vi "Move Motors Y.vi"() -> ()   [LabVIEW 2014]
panel:
  in  "Current Motor Position past home (um)":string
  out "Motor XY After Moving":string
  in  "Camera Resolution X":i64
  in  "pix/micron":dbl
  in  "XY Mouse Position":string
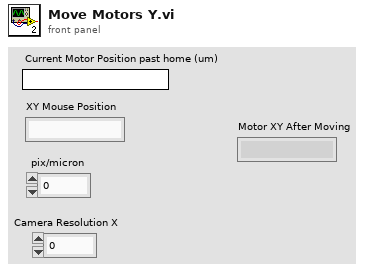
[diagram p1: front panel]
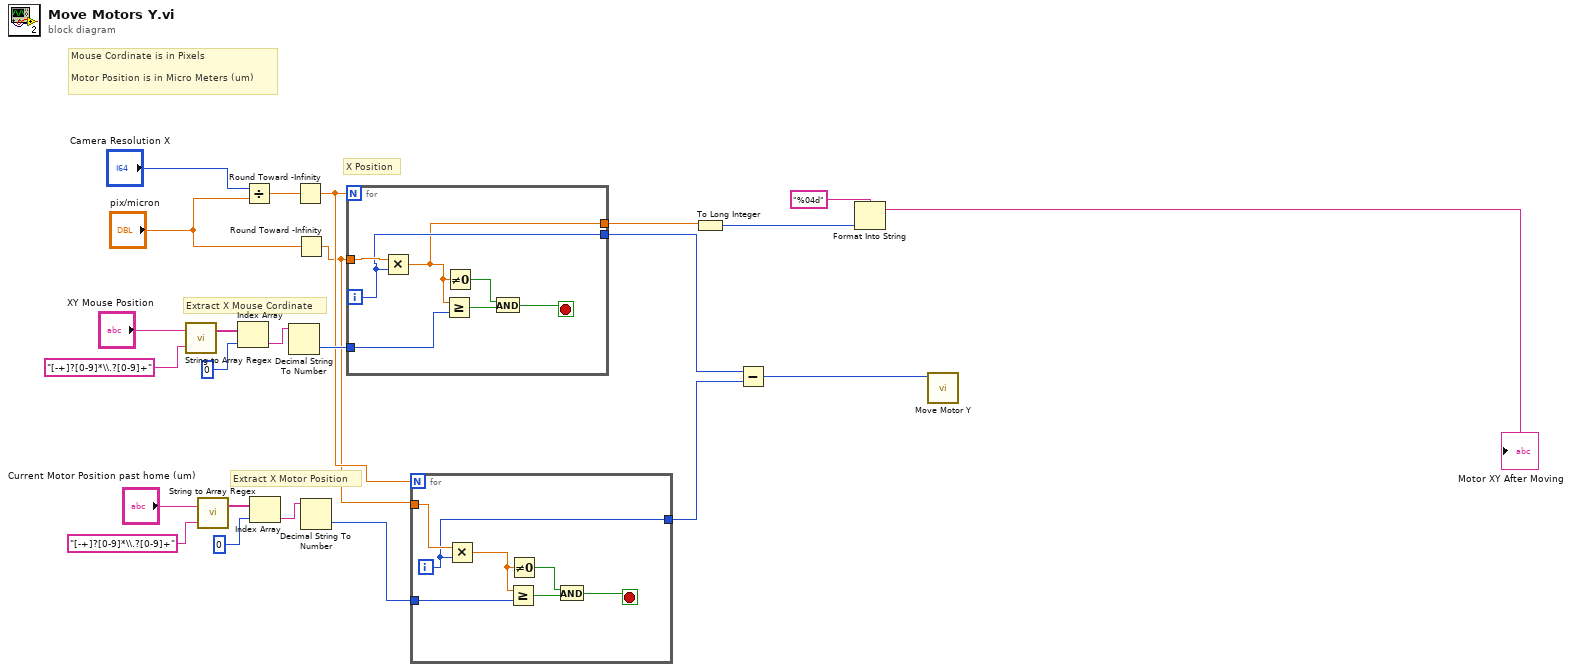
[diagram p0: block diagram]
diagram:
  # "Extract X Motor Position"
  # "Mouse Cordinate is in Pixels\n\nMotor Position is in Micro Meters (um)"
  # "Extract X Mouse Cordinate"
  # "X Position"
  n1 = call "String to Array Regex.vi"("Regex"="[-+]?[0-9]*\\.?[0-9]+", "Message"="XY Mouse Position") -> ("String to Array"=w20:string[])  [unwired: 1 in]
  n2 = call "String to Array Regex.vi"("Regex"="[-+]?[0-9]*\\.?[0-9]+", "Message"="Current Motor Position past home (um)") -> ("String to Array"=w13:string[])  [unwired: 1 in]
  n3 = Index Array(array=w20, index=0) -> (element=w17:string)
  n4 = Divide(x="Camera Resolution X", y="pix/micron") -> (x/y=w23:dbl)
  n5 = Index Array(array=w13, index=0) -> (element=w11:string)
  n6 = Decimal String To Number(string=w17) -> (number=w18:i32)  [unwired: 2 in, 1 out]
  n7 = Round Toward -Infinity(1:w23) -> (0:w8:dbl)
  n8 = Round Toward -Infinity(1:"pix/micron") -> (0:w7:dbl)
  n9 = Decimal String To Number(string=w11) -> (number=w5:i32)  [unwired: 2 in, 1 out]
  n10 = for {
    N: w8 -> [_]
    tunnel: w18 -> [w31]
    tunnel: w7 -> [w28]
    tunnel: [w26] -> w4
    tunnel: [w25] -> w2
    i -> [w26]
    stop <- w27 stop-if-true
    n11 = Multiply(x=w28, y=w26) -> (x*y=w25:dbl)
    n12 = Greater Or Equal?(x=w25, y=w31) -> (x >= y?=w30:bool)
    n13 = Not Equal To 0?(x=w25) -> (x != 0?=w29:bool)
    n14 = And(x=w29, y=w30) -> (x .and. y?=w27:bool)
  }
  n15 = for {
    N: w8 -> [_]
    tunnel: w7 -> [w35]
    tunnel: [w33] -> w6
    tunnel: w5 -> [w32]
    i -> [w33]
    stop <- w36 stop-if-true
    n16 = Multiply(x=w35, y=w33) -> (x*y=w34:dbl)
    n17 = Greater Or Equal?(x=w34, y=w32) -> (x >= y?=w38:bool)
    n18 = Not Equal To 0?(x=w34) -> (x != 0?=w37:bool)
    n19 = And(x=w37, y=w38) -> (x .and. y?=w36:bool)
  }
  n20 = To Long Integer(number=w2) -> (32bit integer=w3:i32)
  n21 = Subtract(x=w4, y=w6) -> (x-y=w1:i32)
  n22 = Format Into String(format string="%04d", w3) -> (resulting string=→"Motor XY After Moving":string)  [unwired: 2 in, 1 out]
  n23 = call "Move Motor Y.vi"("Move X"=w1) -> ()  [unwired: 11 in]
